vi "Link Control References.vi"(8 "error in":errorcluster, 10 "Control Map":T1[](array[typedef]), 11 "PRM in":refnum<class "PRM.lvclass">) -> (0 "error out":errorcluster, 3 "PRM out":refnum<class "PRM.lvclass">)   [LabVIEW 2019, in "PRM.lvlib" / "PRM.lvclass"]
uses:
  Library/PRM.lvclass
  builds/Instruments/Instruments.lvlibp/Library/Instruments.lvclass
  builds/Instruments/Instruments.lvlibp/Custom Controls/Control Element.ctl
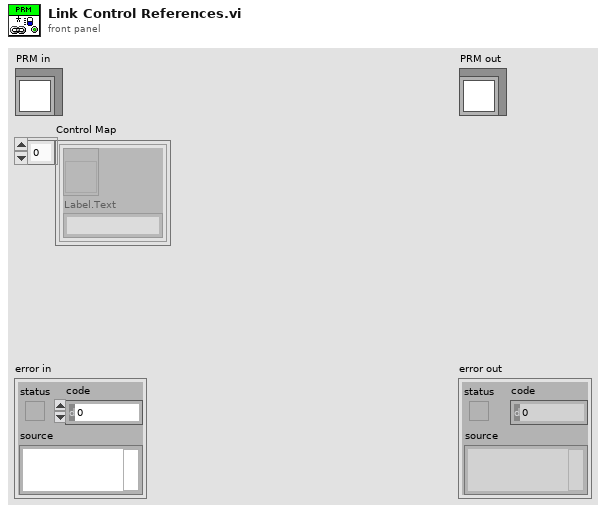
[diagram p1: front panel]
types:
  T1 = typedef "Instruments.lvlibp/Instruments.lvclass/Control Element.ctl" = cluster{refnum<vi>, "Label.Text":string}
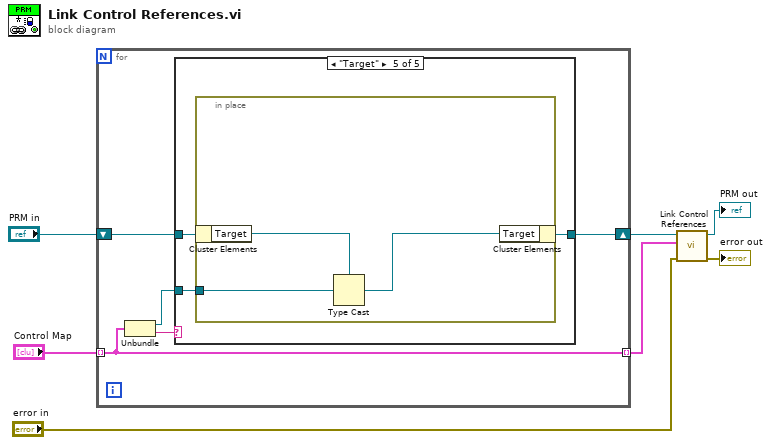
[diagram p0: block diagram]
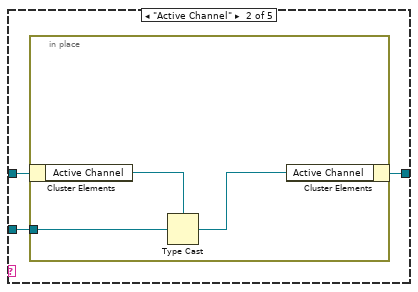
[diagram p3: hidden frame]
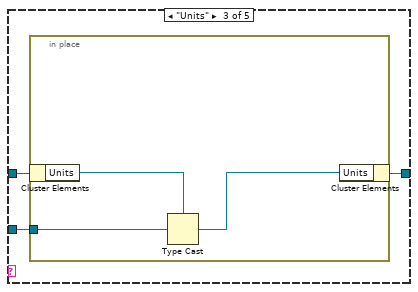
[diagram p4: hidden frame]
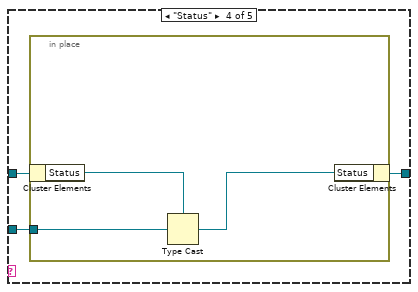
[diagram p5: hidden frame]
diagram:
  n1 = for {
    shift-right: [w8] -> w4
    shift-left: "PRM in" -> [w9]
    tunnel: "Control Map" -> [w12] mode=indexing
    tunnel: [w12] -> w2 mode=indexing
    n2 = Unbundle(w12) -> (w10:refnum<vi>, "Label.Text"=w11:string)
    n3 = case shown="\"Target\"" w11 {
      tunnel: w10 -> [_ w14 w20 w26 w32]
      tunnel: w9 -> [w13 w16 w22 w28 w34]
      tunnel: [w13 w15 w21 w27 w33] -> w8
      frame "False", Default {
      }
      frame "Active Channel" {
        n4 = in-place {
          in-place-border: w14 -> [w18]
          n5 = in-place-cluster #1(w16) -> ("Active Channel"=w19:refnum<vi>)
          n6 = Type Cast(type=w19, x=w18) -> (*(type *) &x=w17:refnum<vi>)
          n7 = in-place-cluster #1("Active Channel"=w17) -> (w15:refnum<class "PRM.lvclass">)
        }
      }
      frame "Units" {
        n8 = in-place {
          in-place-border: w20 -> [w24]
          n9 = in-place-cluster #2(w22) -> ("Units"=w25:refnum<vi>)
          n10 = Type Cast(type=w25, x=w24) -> (*(type *) &x=w23:refnum<vi>)
          n11 = in-place-cluster #2("Units"=w23) -> (w21:refnum<class "PRM.lvclass">)
        }
      }
      frame "Status" {
        n12 = in-place {
          in-place-border: w26 -> [w30]
          n13 = in-place-cluster #3(w28) -> ("Status"=w31:refnum<vi>)
          n14 = Type Cast(type=w31, x=w30) -> (*(type *) &x=w29:refnum<vi>)
          n15 = in-place-cluster #3("Status"=w29) -> (w27:refnum<class "PRM.lvclass">)
        }
      }
      frame "Target" {
        n16 = in-place {
          in-place-border: w32 -> [w36]
          n17 = in-place-cluster #4(w34) -> ("Target"=w37:refnum<vi>)
          n18 = Type Cast(type=w37, x=w36) -> (*(type *) &x=w35:refnum<vi>)
          n19 = in-place-cluster #4("Target"=w35) -> (w33:refnum<class "PRM.lvclass">)
        }
      }
    }
  }
  n20 = call-parent "Link Control References.vi"("error in (no error)"="error in", "Control Map"=w2, "Instruments in"=w4) -> ("error out"=→"error out":errorcluster, "Instruments out"=→"PRM out":refnum<class "PRM.lvclass">)  [unwired: 7 in]
